vi "Example Graph.vi"() -> ()   [LabVIEW 2013]
uses:
  C:/tf/play/labview/Tinkerforge.dll
  Tinkerforge.dll
panel:
  in  "stop":bool
  out "graph":cluster{"z":i32[]}[](graph)
  in  "uid":string="amb"
  in  "port":i32=4223
  in  "host":string="localhost"
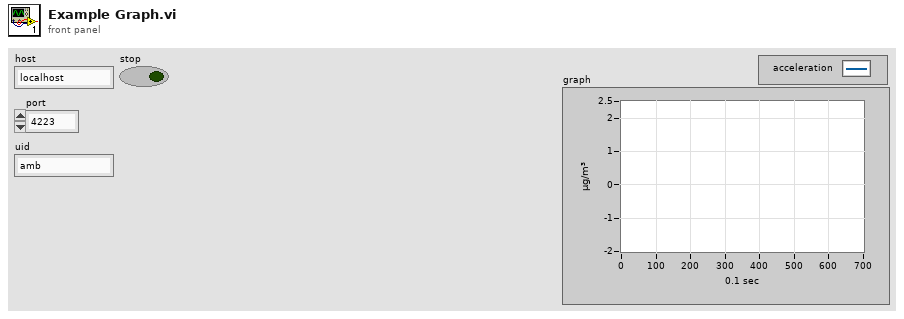
[diagram p1: front panel]
types:
  T1 = cluster{"pm10":i32[], "pm25":i32[], "pm100":i32[]}
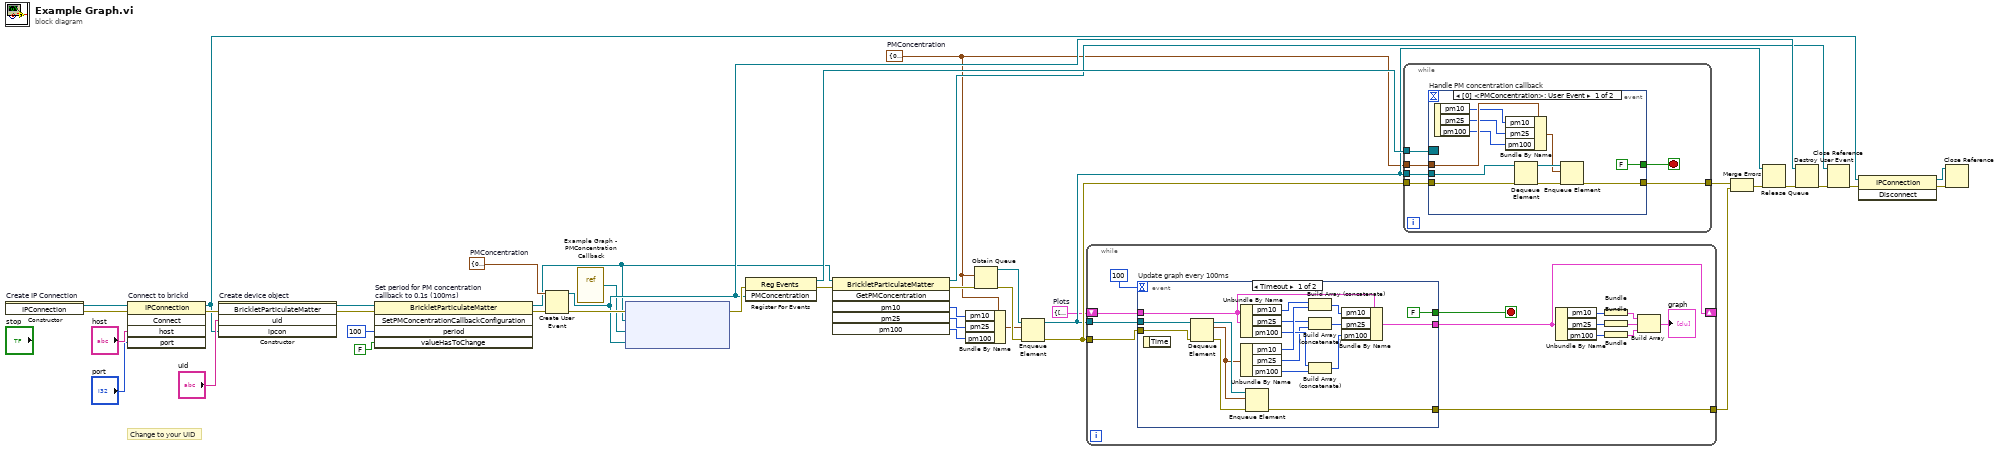
[diagram p0: block diagram]
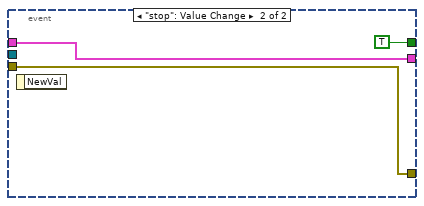
[diagram p2: hidden frame]
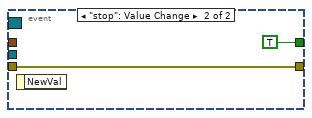
[diagram p3: hidden frame]
diagram:
  w4 = cluster{"pm10":i32, "pm25":i32, "pm100":i32} {"pm10"=0, "pm25"=0, "pm100"=0}  # PMConcentration
  w7 = T1 {"pm10"=[], "pm25"=[], "pm100"=[]}  # Plots
  w26 = cluster{"pm10":i32, "pm25":i32, "pm100":i32} {"pm10"=0, "pm25"=0, "pm100"=0}  # PMConcentration
  # "Change to your UID"
  n1 = constructor on="Create IP Connection" class="IPConnection"() -> (reference out=w40:refnum<k24>, error out=w13:errorcluster)  [unwired: 3 in, 1 out]
  n2 = invoke on="Connect to brickd" class="IPConnection" method="Connect"(reference=w40, error in=w13, "host"="host", "port"="port") -> (reference out=w33:refnum<k24>, error out=w36:errorcluster)  [unwired: 1 in, 3 out]
  n3 = constructor on="Create device object" class="BrickletParticulateMatter"(error in=w36, "uid"="uid", "ipcon"=w33) -> (reference out=w23:refnum<k24>, error out=w25:errorcluster)  [unwired: 2 in, 3 out]
  n4 = invoke on="Set period for PM concentration\ncallback to 0.1s (100ms)" class="BrickletParticulateMatter" method="SetPMConcentrationCallbackConfiguration"(reference=w23, error in=w25, "period"=i64 100, "valueHasToChange"=FALSE) -> (reference out=w10:refnum<k24>, error out=w24:errorcluster)  [unwired: 1 in, 3 out]
  n5 = Create User Event(user event datatype=w26, error in=w24) -> (user event=w28:refnum<user-event>, error out=w31:errorcluster)
  n6 = vi-ref "Example Graph - PMConcentration Callback.vi"() -> ("vi reference"=w5:refnum<vi>)
  n7 = node ("Register Event Callback")(w31, w10, w5, w28) -> (w30:errorcluster)  [unwired: 1 in, 1 out]
  n8 = register-events(error in=w30, w28) -> (reference out=w29:refnum<event-registration>, error out=w12:errorcluster)  [unwired: 1 in]
  n9 = invoke class="BrickletParticulateMatter" method="GetPMConcentration"(reference=w10, error in=w12) -> (reference out=w9:refnum<k24>, error out=w11:errorcluster, "pm10"=w3:i32, "pm25"=w2:i32, "pm100"=w1:i32)  [unwired: 4 in, 1 out]
  n10 = Bundle By Name(cluster=w4, "pm10"=w3, "pm25"=w2, "pm100"=w1) -> (w8:cluster{"pm10":i32, "pm25":i32, "pm100":i32})
  n11 = Obtain Queue(element data type=w4, error in (no error)=w11) -> (queue out=w17:refnum<queue>, error out=w19:errorcluster)  [unwired: 3 in, 1 out]
  n12 = Enqueue Element(queue=w17, element=w8, error in (no error)=w19) -> (queue out=w14:refnum<queue>, error out=w18:errorcluster)  [unwired: 1 in, 1 out]
  n13 = while {
    tunnel: [w51] -> w21
    tunnel: w18 -> [w52]
    shift-right: [w48] -> _
    shift-left: w7 -> [w53]
    tunnel: w14 -> [w50]
    stop <- w49 stop-if-true
    n14 = event "Update graph every 100ms" shown="[0] Timeout" {
      selector: _ -> [_ _]
      dyn-events: _ -> [_ _]
      timeout: 100 -> [_ _]
      tunnel: [w64 w74] -> w48
      tunnel: w53 -> [w65 w74]
      tunnel: w52 -> [w72 w73]
      tunnel: [w69 w73] -> w51
      tunnel: w50 -> [w71 _]
      tunnel: [FALSE TRUE] -> w49
      event Timeout {
        n15 = event-data() -> ()  [unwired: 1 in, 1 out]
        n16 = Dequeue Element(queue=w71, error in (no error)=w72) -> (queue out=w68:refnum<queue>, element=w66:cluster{"pm10":i32, "pm25":i32, "pm100":i32}, error out=w70:errorcluster)  [unwired: 1 in, 1 out]
        n17 = Unbundle By Name(w65) -> ("pm10"=w63:i32[], "pm25"=w60:i32[], "pm100"=w57:i32[])
        n18 = Unbundle By Name(w66) -> ("pm10"=w62:i32, "pm25"=w56:i32, "pm100"=w55:i32)
        n19 = Enqueue Element(queue=w68, element=w66, error in (no error)=w70) -> (error out=w69:errorcluster)  [unwired: 1 in, 2 out]
        n20 = Build Array (concatenate)(w63, w62) -> (w61:i32[])
        n21 = Build Array (concatenate)(w60, w56) -> (w59:i32[])
        n22 = Build Array (concatenate)(w57, w55) -> (w58:i32[])
        n23 = Bundle By Name(cluster=w65, "pm10"=w61, "pm25"=w59, "pm100"=w58) -> (w64:T1)
      }
      event "stop": Value Change {
        n24 = event-data() -> ()  [unwired: 1 in, 1 out]
      }
    }
    n25 = Unbundle By Name(w48) -> ("pm10"=w47:i32[], "pm25"=w45:i32[], "pm100"=w43:i32[])
    n26 = Bundle("pm10"=w47) -> (w46:cluster{"pm10":i32[]})  [unwired: 1 in]
    n27 = Bundle("pm25"=w45) -> (w44:cluster{"pm25":i32[]})  [unwired: 1 in]
    n28 = Bundle("pm100"=w43) -> (w42:cluster{"pm100":i32[]})  [unwired: 1 in]
    n29 = Build Array(w46, w44, w42) -> (→"graph":cluster{"pm100":i32[]}[])
  }
  n30 = while {
    tunnel: w29 -> [w81]
    tunnel: [w79] -> w20
    tunnel: w18 -> [w80]
    tunnel: w14 -> [w78]
    tunnel: w4 -> [w76]
    stop <- w77 stop-if-true
    n31 = event "Handle PM concentration callback" shown="[0] <PMConcentration>: User Event" {
      selector: w81 -> [_ _]
      dyn-events: _ -> [_ _]
      timeout: _ -> [_ _]
      tunnel: w80 -> [w92 w93]
      tunnel: [w90 w93] -> w79
      tunnel: w78 -> [w89 _]
      tunnel: [FALSE TRUE] -> w77
      tunnel: w76 -> [w85 _]
      event User Event {
        n32 = event-data() -> ("pm10"=w84:i32, "pm25"=w83:i32, "pm100"=w82:i32)  [unwired: 1 in]
        n33 = Bundle By Name(cluster=w85, "pm10"=w84, "pm25"=w83, "pm100"=w82) -> (w86:cluster{"pm10":i32, "pm25":i32, "pm100":i32})
        n34 = Dequeue Element(queue=w89, error in (no error)=w92) -> (queue out=w88:refnum<queue>, error out=w91:errorcluster)  [unwired: 1 in, 2 out]
        n35 = Enqueue Element(queue=w88, element=w86, error in (no error)=w91) -> (error out=w90:errorcluster)  [unwired: 1 in, 2 out]
      }
      event "stop": Value Change {
        n36 = event-data() -> ()  [unwired: 1 in, 1 out]
      }
    }
  }
  n37 = Merge Errors(w20, w21) -> (w16:errorcluster)
  n38 = Release Queue(queue=w14, error in (no error)=w16) -> (error out=w15:errorcluster)  [unwired: 1 in, 2 out]
  n39 = Destroy User Event(user event=w28, error in=w15) -> (error out=w27:errorcluster)
  n40 = Close Reference(reference=w9, error in (no error)=w27) -> (error out=w35:errorcluster)
  n41 = invoke class="IPConnection" method="Disconnect"(reference=w33, error in=w35) -> (reference out=w32:refnum<k24>, error out=w34:errorcluster)  [unwired: 1 in, 1 out]
  n42 = Close Reference(reference=w32, error in (no error)=w34) -> ()  [unwired: 1 out]
